vi "Render Inverted Section with Boolean False Pair.vi"(8 "Error In":errorcluster) -> (0 "Error Out":errorcluster)   [LabVIEW 2018, in "Tests.lvlib" / "Render.lvlib"]
uses:
  Render.lvlib
  src/Toolkit/Data/Pair/Pair.lvclass
  D:/Users/cfield/Code/Field R&D Services/Labstache/src/Toolkit/Data/Datum/Datum.lvclass
  src/Toolkit/Data/Pair/Support/From Boolean.vi
  src/Toolkit/Low-Level/Renderer/Renderer.lvclass
  <vilib>/addons/_JKI Toolkits/Caraya/classes/Test/Test.lvclass
  <vilib>/addons/_JKI Toolkits/Caraya/classes/Assert/Assert.lvclass
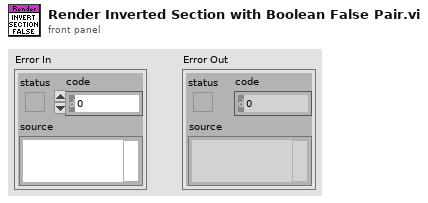
[diagram p1: front panel]
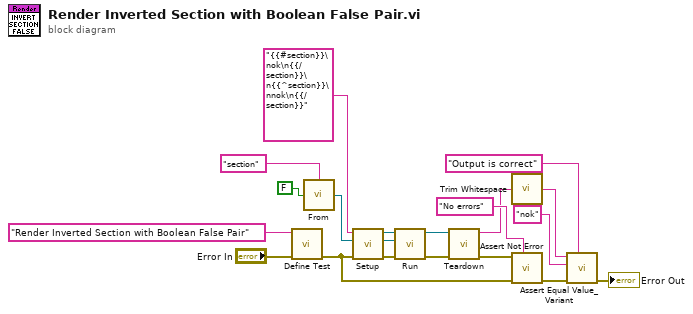
[diagram p0: block diagram]
diagram:
  n1 = call <vilib>:"Define Test.vi"("error in (no error)"="Error In", "Label (VI Title)"="Render Inverted Section with Boolean False Pair") -> ("error out"=w12:errorcluster)  [unwired: 9 in]
  n2 = call-poly "From.vi"("Value"=FALSE, "Key"="section") -> ("Pair"=w2:refnum<class "Pair.lvclass">)
  n3 = call "Setup.vi"("Error In"=w12, "Data"=w2, "Value"="{{#section}}\nok\n{{/section}}\n{{^section}}\nnok\n{{/section}}" ("Input")) -> ("Error Out"=w13:errorcluster, "Abstract Syntax Tree"=w1:refnum<class "Root.lvclass">, "Renderer"=w14:refnum<class "Renderer.lvclass">)  [unwired: 6 in]
  n4 = call-dynamic "Run.vi"("Error In"=w13, "Abstract Syntax Tree"=w1, "Renderer In"=w14) -> ("Error Out"=w6:errorcluster, "Renderer Out"=w3:refnum<class "Renderer.lvclass">)  [unwired: 7 in]
  n5 = call "Teardown.vi"("Error In"=w6, "Renderer"=w3) -> ("Error Out"=w5:errorcluster, "Output"=w4:string)  [unwired: 8 in]
  n6 = call <vilib>:"Trim Whitespace.vi"("string"=w4) -> ("trimmed string"=w9:string)  [unwired: 1 in]
  n7 = call <vilib>:"Assert Not Error.vi"("Label"="No errors", "error in (no error)"=w12, "Not Error?"=w5) -> ("error out"=w17:errorcluster)  [unwired: 8 in]
  n8 = call <vilib>:"Assert Equal Value_Variant.vi"("Label"="Output is correct", "error in (no error)"=w17, "Y"="nok", "X"=w9) -> ("error out"=→"Error Out":errorcluster)  [unwired: 7 in]
